vi "Waveform Data Analysis.vi"(8 "error in (no error)":errorcluster, 11 "Waveform data":dbl[](array[numeric])) -> (0 "error out":errorcluster, 1 "first sample":dbl, 3 "Waveform data dup":dbl[](array[numeric]), 4 "mean":dbl, 6 "last sample":dbl)   [LabVIEW 2013, in "Waveforms Generation Custom Device.lvlib"]
uses:
  Waveforms Generation Custom Device.lvlib
  <vilib>/Analysis/baseanly.llb/Mean (DBL).vi
  <vilib>/Analysis/NI_AALBase.lvlib
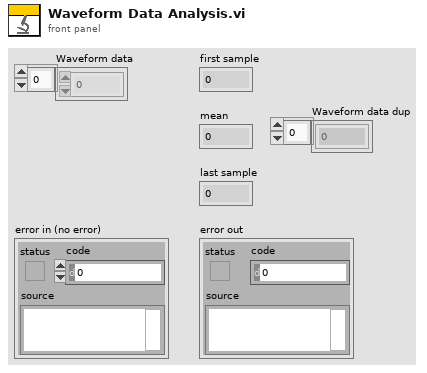
[diagram p1: front panel]
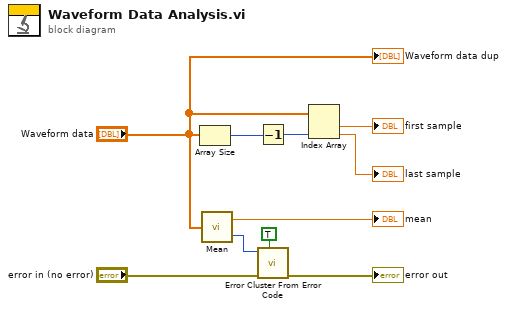
[diagram p0: block diagram]
diagram:
  n1 = Array Size(array="Waveform data") -> (size(s)=w2:i32)
  n2 = call-poly <vilib>:"Mean.vi"("X"="Waveform data") -> ("mean"=→"mean":dbl, "error"=w5:i32)
  n3 = Decrement(x=w2) -> (x-1=w3:i32)
  n4 = call <vilib>:"Error Cluster From Error Code.vi"("show call chain? (False)"=TRUE, "error in (no error)"="error in (no error)", "error code (0)"=w5) -> ("error out"=→"error out":errorcluster)  [unwired: 6 in]
  n5 = Index Array(array="Waveform data", index #2=w3) -> (element #1=→"first sample":dbl, element #2=→"last sample":dbl)  [unwired: 1 in]
  "Waveform data dup" <- "Waveform data"
